vi "PMX_GetLimitSwitch.vi"(8 "Error in":errorcluster, 10 "LimitSwitchNumber":i32, 11 "Device":refnum<k24>) -> (0 "Error out":errorcluster, 2 "LimitSwitch":T1, 3 "Device":refnum<k24>)   [LabVIEW 2016]
doc: "Gets the limit switch info of the given limit switch number\n\nLimitSwitchNumber: Number of the limit to query (1..32)\nLimitSwitch:\nEnabled: Determines if limit switch operation is activated. \nHysteresis:Hysteresis value. Dependents on OperationDirection, it may also be used to define the band span. \nIgnoreMeasurementValueStatus: Determines if the status of the measurement value is ignored during evaluation of limit switch status.\nInputSignal: Signal whose measurement value is used to evaluate the limit switch. \nInvertResetBehaviour: If true, the defined ResetBehavior is inverted. \nLimit: Limit value. Dependents on OperationDirection, it may also be used to define the lower band value. \nLimitSwitchNumber: Number of the limit switch. This can range from 1 to 32. \nOperatingDirection: Operation direction of the limit switch. \nResetBehaviorMask: Reset behavior. Binary mask which is ANDed with all digital inputs. The reset behavior can be inverted with InvertResetBehavior. Default setting is 0."
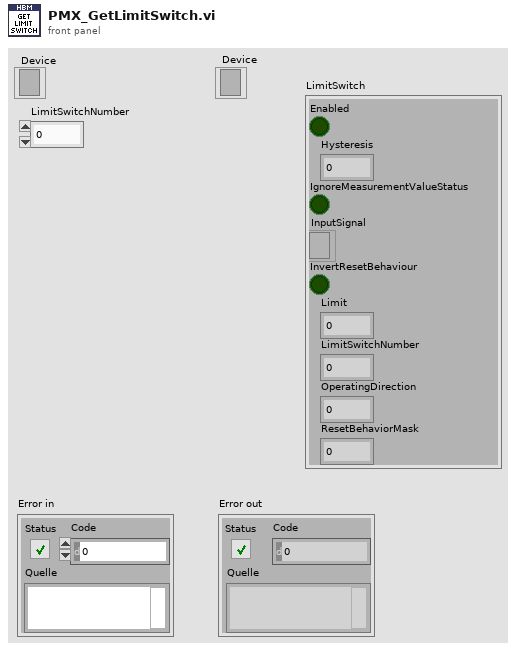
[diagram p1: front panel]
types:
  T1 = cluster{"Enabled":bool, "Hysteresis":dbl, "IgnoreMeasurementValueStatus":bool, "InputSignal":refnum<k24>, "InvertResetBehaviour":bool, "Limit":dbl, "LimitSwitchNumber":i32, "OperatingDirection":i32, "ResetBehaviorMask":i32}
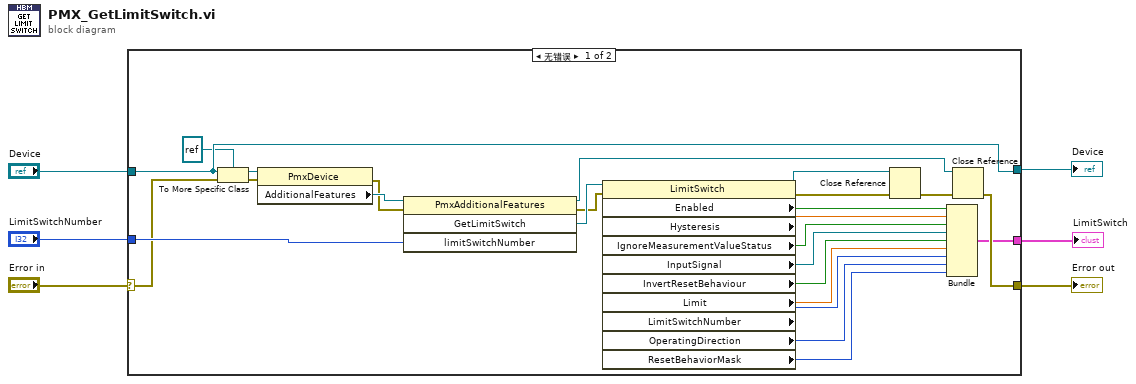
[diagram p0: block diagram]
diagram:
  n1 = case shown="无错误" "Error in" {
    selector: "Error in" -> [w15 w33]
    tunnel: [w11 w33] -> w4
    tunnel: "Device" -> [w26 w32]
    tunnel: [w26 w32] -> w5
    tunnel: "LimitSwitchNumber" -> [w27 _]
    tunnel: [w9 _] -> w1
    frame No Error {
      n2 = To More Specific Class(target class=refnum<k24> refnum ("Zielklasse"), reference=w26, error in=w15) -> (specific class reference=w31:refnum<k24>, error out=w28:errorcluster)
      n3 = property on="Eigenschaftsknoten" class="PmxDevice"(reference=w31, error in=w28) -> (error out=w29:errorcluster, "AdditionalFeatures"=w30:refnum<k24>)  [unwired: 1 out]
      n4 = invoke on="Methodenknoten" class="PmxAdditionalFeatures" method="GetLimitSwitch"(reference=w30, error in=w29, "limitSwitchNumber"=w27) -> (reference out=w12:refnum<k24>, error out=w24:errorcluster, "GetLimitSwitch"=w25:refnum<k24>)  [unwired: 1 in, 1 out]
      n5 = property on="Eigenschaftsknoten" class="LimitSwitch"(reference=w25, error in=w24) -> (reference out=w10:refnum<k24>, error out=w7:errorcluster, "Enabled"=w23:bool, "Hysteresis"=w22:dbl, "IgnoreMeasurementValueStatus"=w21:bool, "InputSignal"=w8:refnum<k24>, "InvertResetBehaviour"=w20:bool, "Limit"=w19:dbl, "LimitSwitchNumber"=w18:i32, "OperatingDirection"=w17:i32, "ResetBehaviorMask"=w16:i32)
      n6 = Close Reference(reference=w10, error in (no error)=w7) -> (error out=w13:errorcluster)
      n7 = Bundle("Enabled"=w23, "Hysteresis"=w22, "IgnoreMeasurementValueStatus"=w21, "InputSignal"=w8, "InvertResetBehaviour"=w20, "Limit"=w19, "LimitSwitchNumber"=w18, "OperatingDirection"=w17, "ResetBehaviorMask"=w16) -> (w9:T1)  [unwired: 1 in]
      n8 = Close Reference(reference=w12, error in (no error)=w13) -> (error out=w11:errorcluster)
    }
    frame Error {
    }
  }
  "Device" <- w5
  "Error out" <- w4
  "LimitSwitch" <- w1
